vi "datalogger.vi"(8 "File ref":refnum<file>, 9 "data log interval (s)":u32=1 min=1, 10 "Plant State":T3=1 items=["OFF"], 11 "Sensor Data":T1 {"Sensor array"."scaled" format="%.2f"; "Sensor array"."voltage" format="%.4f"; "Time" format="%<%I:%M:%S%2u %p\n%m/%d/%Y>T"}) -> (3 "Sensor Data out":T1 {"Sensor array"."scaled" format="%.2f"; "Sensor array"."voltage" format="%.4f"; "Time" format="%<%I:%M:%S%2u %p\n%m/%d/%Y>T"})   [LabVIEW 2010]
uses:
  calibration/global scale array.vi
  DAQ configuration/sensor cluster.ctl
  TCP DAQ/Sensor data.ctl
  Process Controller 3.0/Plant state.ctl
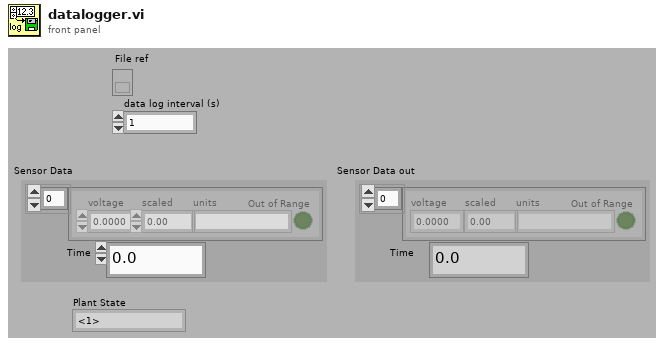
[diagram p1: front panel]
types:
  T1 = typedef "Sensor data.ctl" = cluster{" Sensor array":T2[], "Time":dbl}
  T2 = typedef "sensor cluster.ctl" = cluster{"voltage":sgl, "scaled":sgl, "units":string, "Out of Range":bool}
  T3 = typedef "Plant state.ctl" = u16
  T4 = typedef "calib array.ctl" = T5[]
  T5 = typedef "conversion.ctl" = cluster{"conversion matrix":sgl[][], "units":string, "name":string, "scale type":T6, "offset (volts)":dbl, "second channel":i8, "correspondence table":T7, "offset (physical units)":dbl, "pH scale":T8, "D.O.":T9}
  T6 = typedef "scale type.ctl" = enum16{"Volts", "Polynomial", "Correspondence Table", "pH", "Dissolved Oxygen", "Quadratic"}
  T7 = typedef "correspondence table.ctl" = cluster{"physical units":dbl, "volts":dbl}[]
  T8 = typedef "pH scale.ctl" = cluster{"Buffers":cluster{"Buffer":dbl, "Calibrated":bool, "V/T":dbl}[], "Temperature":dbl}
  T9 = typedef "DO scale.ctl" = cluster{"Temperature":dbl, "K":dbl, "barometric pressure":dbl}
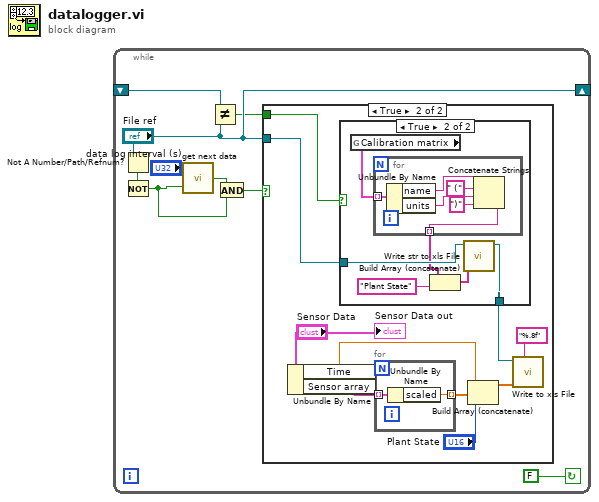
[diagram p0: block diagram]
diagram:
  n1 = while {
    shift-left: _ -> [w7]
    shift-right: ["File ref"] -> _
    stop <- FALSE continue-if-true
    n2 = Not A Number/Path/Refnum?(number/path/refnum="File ref") -> (NaN/Path/Refnum?=w8:bool)
    n3 = Not(x=w8) -> (.not. x?=w3:bool)
    n4 = call "get next data.vi"("Monitor Data"=w3, "data interval (s)"="data log interval (s)") -> ("get next"=w2:bool)
    n5 = Not Equal?(x=w7, y="File ref") -> (x != y?=w5:bool)
    n6 = And(x=w2, y=w3) -> (x .and. y?=w1:bool)
    n7 = case shown="True" w1 {
      tunnel: "File ref" -> [_ w12]
      tunnel: w5 -> [_ w14]
      frame False {
      }
      frame True {
        n8 = Unbundle By Name("Sensor Data") -> ("Time"=w11:dbl, "Sensor array"=w17:T2[])
        n9 = case shown="True" w14 {
          tunnel: w12 -> [w20 w26]
          tunnel: [w20 w25] -> w13
          frame False {
          }
          frame True {
            n10 = global read "global scale array.vi" "Calibration matrix"() -> (w24:T4)
            n11 = for {
              tunnel: w24 -> [w32] mode=indexing
              tunnel: [w27] -> w23 mode=indexing
              n12 = Unbundle By Name(w32) -> ("name"=w31:string, "units"=w29:string)
              n13 = Concatenate Strings(w31, " (" ("Substring"), w29, ")" ("Substring")) -> (w27:string)
            }
            n14 = Build Array (concatenate)(w23, "Plant State" ("Substring")) -> (w22:string[])
            n15 = call "Write str to xls File.vi"("error in (no error)"=w22, "refnum"=w26) -> ("dup refnum"=w25:refnum<file>)  [unwired: 8 in, 1 out]
          }
        }
        n16 = for {
          tunnel: w17 -> [w34] mode=indexing
          tunnel: [w33] -> w16 mode=indexing
          n17 = Unbundle By Name(w34) -> ("scaled"=w33:sgl)
        }
        n18 = Build Array (concatenate)(w11, w16, "Plant State") -> (w15:dbl[])
        n19 = call "Write to xls File.vi"("format (%.3f)"="%.8f", "error in (no error)"=w15, "refnum"=w13) -> ()  [unwired: 7 in, 2 out]
        "Sensor Data out" <- "Sensor Data"
      }
    }
  }
